vi "F_envelope.vi"(5 "XY_in":cluster{"S":dbl[], "F":dbl[]}, 9 "limit":T2) -> (6 "XY_out":cluster{dbl[], dbl[]}[](graph), 10 "ok":bool, 14 "interval_data_parameter":T1(array[cluster]), 15 "ok_all interval":bool[](array[boolean]))   [LabVIEW 2017]
panel:
  # "每个区间数据及区间范围"
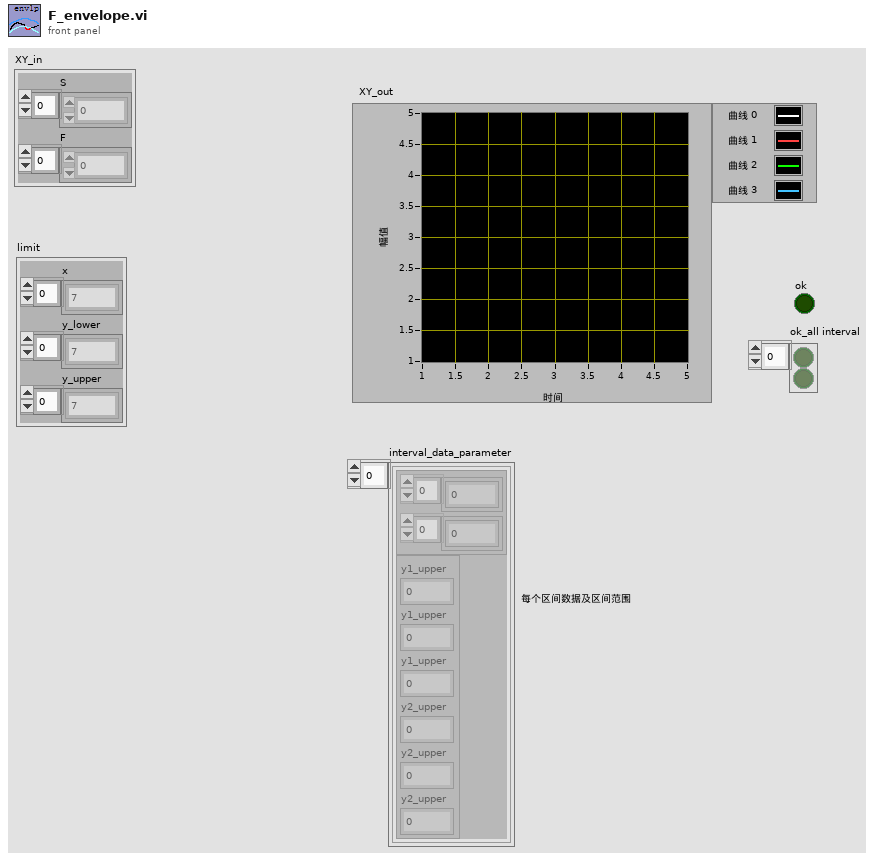
[diagram p1: front panel]
types:
  T1 = cluster{cluster{dbl[], dbl[]}, cluster{"y1_upper":dbl, "y1_upper":dbl, "y1_upper":dbl, "y2_upper":dbl, "y2_upper":dbl, "y2_upper":dbl}}[]
  T2 = cluster{"x":dbl[], "y_lower":dbl[], "y_upper":dbl[]}
  T3 = cluster{"y2_upper":dbl, "y2_upper":dbl, "y2_upper":dbl, "y2_upper":dbl, "y2_upper":dbl, "y2_upper":dbl}
  T4 = cluster{cluster{dbl[], dbl[]}, cluster{"y2_upper":dbl, "y2_upper":dbl, "y2_upper":dbl, "y2_upper":dbl, "y2_upper":dbl, "y2_upper":dbl}}
  T5 = cluster{cluster{dbl[], dbl[]}, cluster{"y2_upper":dbl, "y2_upper":dbl, "y2_upper":dbl, "y2_upper":dbl, "y2_upper":dbl, "y2_upper":dbl}}[]
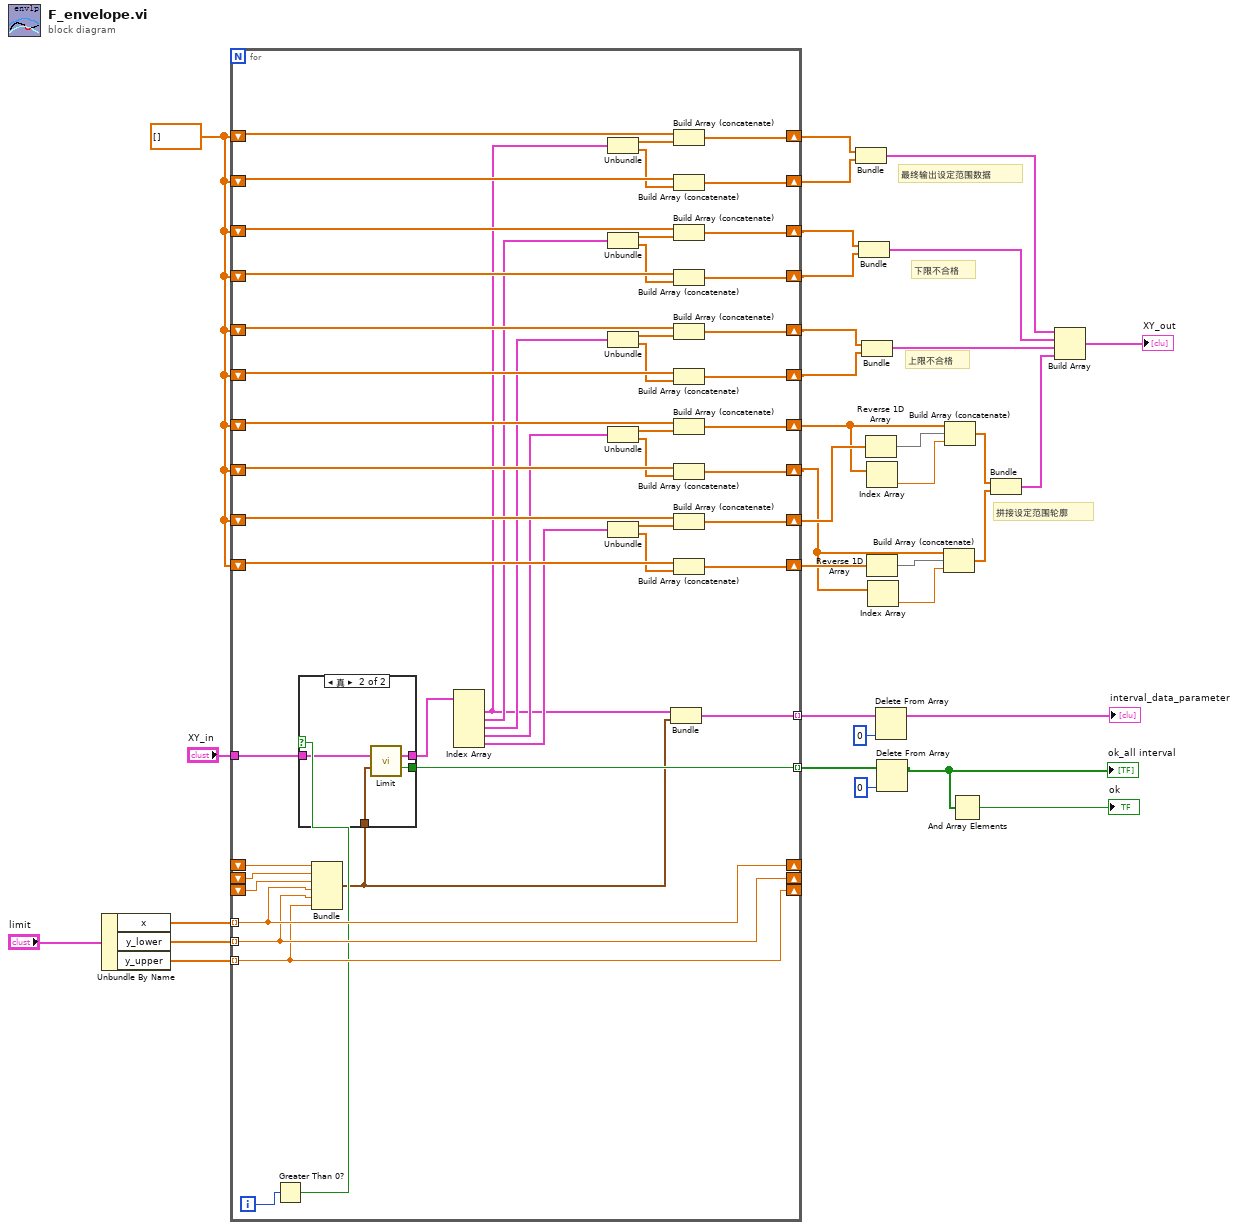
[diagram p0: block diagram]
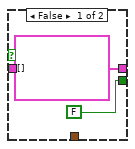
[diagram p2: hidden frame]
diagram:
  w1 = dbl[] []
  # "上限不合格"
  # "下限不合格"
  # "最终输出设定范围数据"
  # "拼接设定范围轮廓"
  n1 = Unbundle By Name("limit") -> ("x"=w33:dbl[], "y_lower"=w32:dbl[], "y_upper"=w31:dbl[])
  n2 = for {
    tunnel: "XY_in" -> [w82]
    tunnel: w33 -> [w42] mode=indexing
    tunnel: w32 -> [w41] mode=indexing
    tunnel: w31 -> [w40] mode=indexing
    shift-right: [w76] -> w12
    shift-left: w1 -> [w77]
    shift-right: [w80] -> w14
    shift-left: w1 -> [w79]
    shift-right: [w66] -> w9
    shift-left: w1 -> [w67]
    shift-right: [w70] -> w10
    shift-left: w1 -> [w69]
    shift-right: [w75] -> w25
    shift-left: w1 -> [w74]
    shift-right: [w71] -> w26
    shift-left: w1 -> [w72]
    shift-right: [w65] -> w27
    shift-left: w1 -> [w64]
    shift-right: [w61] -> w28
    shift-left: w1 -> [w62]
    shift-right: [w56] -> w29
    shift-left: w1 -> [w57]
    shift-right: [w60] -> w30
    shift-left: w1 -> [w59]
    tunnel: [w46] -> w19 mode=indexing
    shift-right: [w42] -> _
    shift-left: _ -> [w45]
    shift-right: [w41] -> _
    shift-left: _ -> [w44]
    shift-right: [w40] -> _
    shift-left: _ -> [w43]
    tunnel: [w36] -> w4 mode=indexing
    i -> [w39]
    n3 = Greater Than 0?(x=w39) -> (x > 0?=w38:bool)
    n4 = Bundle("y2_upper"=w45, "y2_upper"=w44, "y2_upper"=w43, "y2_upper"=w42, "y2_upper"=w41, "y2_upper"=w40) -> (w35:T3)  [unwired: 1 in]
    n5 = case shown="真" w38 {
      tunnel: w82 -> [_ w88]
      tunnel: w35 -> [_ w85]
      tunnel: [cluster{dbl[], dbl[]}[] [] ("XY_out") w87] -> w81
      tunnel: [FALSE ("ok") w86] -> w46
      frame False {
      }
      frame True {
        n6 = call "Limit.vi"("XY_in"=w88, "边界配置"=w85) -> ("XY_out"=w87:cluster{dbl[], dbl[]}[], "ok"=w86:bool)  [unwired: 12 in]
      }
    }
    n7 = Index Array(array=w81) -> (element #1=w37:cluster{dbl[], dbl[]}, element #2=w50:cluster{dbl[], dbl[]}, element #3=w49:cluster{dbl[], dbl[]}, element #4=w48:cluster{dbl[], dbl[]}, element #5=w47:cluster{dbl[], dbl[]})  [unwired: 5 in]
    n8 = Unbundle(w37) -> (w58:dbl[], w55:dbl[])
    n9 = Unbundle(w50) -> (w63:dbl[], w54:dbl[])
    n10 = Unbundle(w49) -> (w73:dbl[], w53:dbl[])
    n11 = Unbundle(w48) -> (w68:dbl[], w52:dbl[])
    n12 = Unbundle(w47) -> (w78:dbl[], w51:dbl[])
    n13 = Bundle(w37, w35) -> (w36:T4)  [unwired: 1 in]
    n14 = Build Array (concatenate)(w59, w58) -> (w60:dbl[])
    n15 = Build Array (concatenate)(w57, w55) -> (w56:dbl[])
    n16 = Build Array (concatenate)(w62, w63) -> (w61:dbl[])
    n17 = Build Array (concatenate)(w64, w54) -> (w65:dbl[])
    n18 = Build Array (concatenate)(w72, w73) -> (w71:dbl[])
    n19 = Build Array (concatenate)(w74, w53) -> (w75:dbl[])
    n20 = Build Array (concatenate)(w69, w68) -> (w70:dbl[])
    n21 = Build Array (concatenate)(w67, w52) -> (w66:dbl[])
    n22 = Build Array (concatenate)(w79, w78) -> (w80:dbl[])
    n23 = Build Array (concatenate)(w77, w51) -> (w76:dbl[])
  }
  n24 = Bundle(w30, w29) -> (w24:cluster{dbl[], dbl[]})  [unwired: 1 in]
  n25 = Bundle(w28, w27) -> (w23:cluster{dbl[], dbl[]})  [unwired: 1 in]
  n26 = Bundle(w26, w25) -> (w22:cluster{dbl[], dbl[]})  [unwired: 1 in]
  n27 = Reverse 1D Array(array=w14) -> (reversed array=w13:dbl[])
  n28 = Index Array(array=w10) -> (element=w8:dbl)  [unwired: 1 in]
  n29 = Reverse 1D Array(array=w12) -> (reversed array=w11:dbl[])
  n30 = Index Array(array=w9) -> (element=w7:dbl)  [unwired: 1 in]
  n31 = Delete From Array(array=w4, index=0 ("索引")) -> (array with subset deleted=→"interval_data_parameter":T5)  [unwired: 1 in, 1 out]
  n32 = Delete From Array(array=w19, index=0 ("索引")) -> (array with subset deleted=w18:bool[])  [unwired: 1 in, 1 out]
  "ok_all interval" <- w18
  n33 = Build Array (concatenate)(w9, w11, w7) -> (w15:dbl[])
  n34 = Build Array (concatenate)(w10, w13, w8) -> (w16:dbl[])
  n35 = And Array Elements(Boolean array=w18) -> (logical AND=→"ok":bool)
  n36 = Bundle(w16, w15) -> (w6:cluster{dbl[], dbl[]})  [unwired: 1 in]
  n37 = Build Array(w24, w23, w22, w6) -> (→"XY_out":cluster{dbl[], dbl[]}[])
